vi "Configure Interpolation.vi"(7 "Enable Display Interpolation (T: Enable)":bool=TRUE, 8 "error in (no error)":errorcluster, 9 "Enable Rise Fall Edges (T: Enable)":bool=TRUE, 10 "Enable Fast Interpolation (T: Enable)":bool=TRUE, 11 "VISA resource name":refnum<visa-resource-name>) -> (0 "error out":errorcluster, 3 "VISA resource name out":refnum<visa-resource-name>)   [LabVIEW 2014, in "Stanford Research SR1.lvlib"]
doc: "Configures the attributes of Interpolation."
uses:
  Stanford Research SR1.lvlib
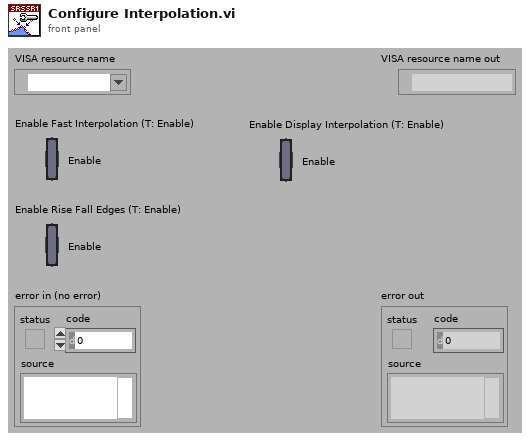
[diagram p1: front panel]
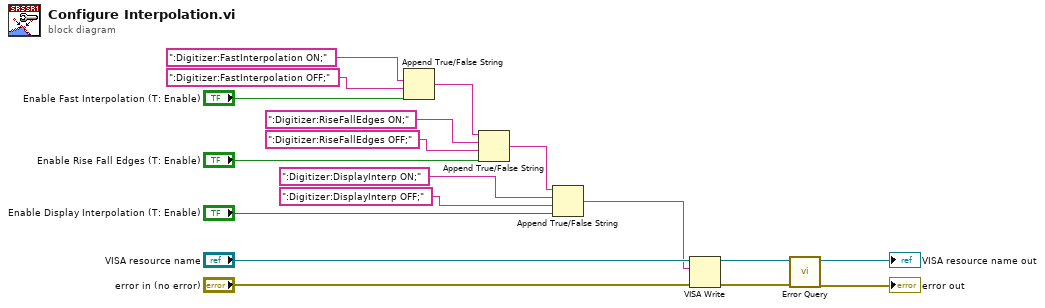
[diagram p0: block diagram]
diagram:
  n1 = Append True/False String(1:"Enable Fast Interpolation (T: Enable)", 2:":Digitizer:FastInterpolation OFF;", 3:":Digitizer:FastInterpolation ON;") -> (0:w15:string)  [unwired: 1 in]
  n2 = Append True/False String(1:"Enable Rise Fall Edges (T: Enable)", 2:":Digitizer:RiseFallEdges OFF;", 3:":Digitizer:RiseFallEdges ON;", 4:w15) -> (0:w2:string)
  n3 = Append True/False String(1:"Enable Display Interpolation (T: Enable)", 2:":Digitizer:DisplayInterp OFF;", 3:":Digitizer:DisplayInterp ON;", 4:w2) -> (0:w3:string)
  n4 = VISA Write(VISA resource name="VISA resource name", write buffer=w3, error in (no error)="error in (no error)") -> (VISA resource name out=w9:refnum<visa-resource-name>, error out=w8:errorcluster)  [unwired: 1 out]
  n5 = call "Error Query.vi"("error in (no error)"=w8, "VISA resource name"=w9) -> ("error out"=→"error out":errorcluster, "VISA resource name out"=→"VISA resource name out":refnum<visa-resource-name>)  [unwired: 6 in, 2 out]
